vi "Example3.vi"() -> ()   [LabVIEW 2020]
doc: "Example of using propety node by direct and by reference."
panel:
  in  "stop":bool
  in  "Range":i32=2 format="%_1f"
  out "XY Graph":cluster{dbl[], dbl[]}[](graph)
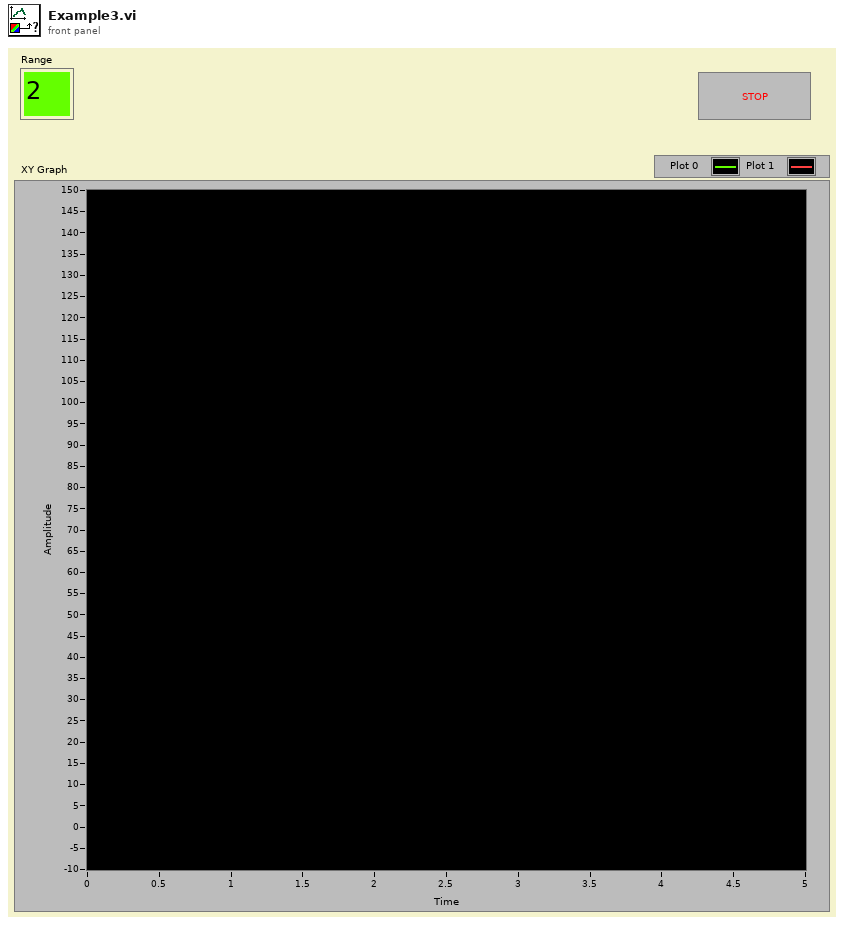
[diagram p1: front panel]
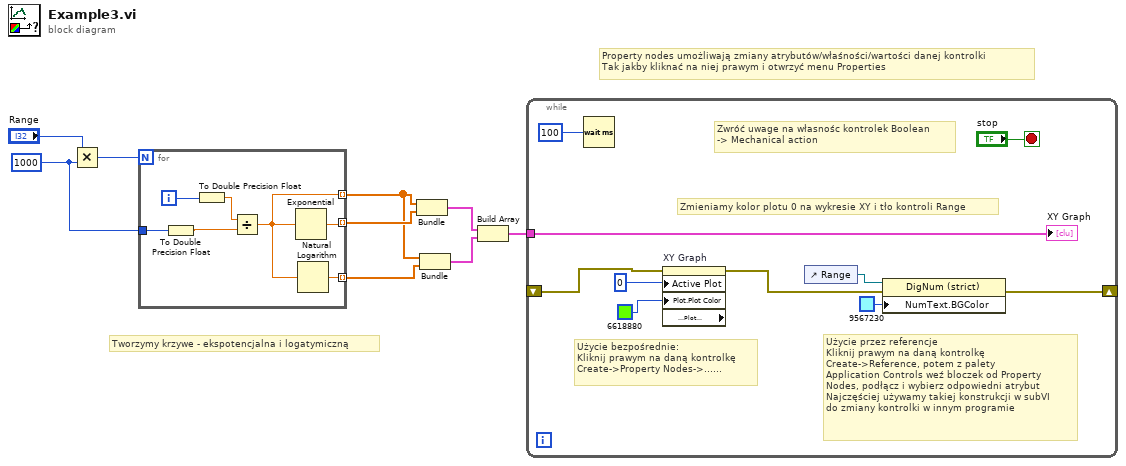
[diagram p0: block diagram]
diagram:
  w3 = 1000
  # "Tworzymy krzywe - ekspotencjalna i logatymiczną"
  # "Property nodes umożliwają zmiany atrybutów/właśności/wartości danej kontrolki \nTak jakby kliknać na niej prawym i otwrzyć menu Properties"
  n1 = Multiply(x="Range", y=w3) -> (x*y=w1:i32)
  n2 = for {
    N: w1 -> [_]
    tunnel: [w15] -> w9 mode=indexing
    tunnel: [w14] -> w8 mode=indexing
    tunnel: [w13] -> w7 mode=indexing
    tunnel: w3 -> [w11]
    i -> [w12]
    n3 = To Double Precision Float(number=w11) -> (double precision float=w10:dbl)
    n4 = To Double Precision Float(number=w12) -> (double precision float=w16:dbl)
    n5 = Divide(x=w16, y=w10) -> (x/y=w14:dbl)
    n6 = Exponential(1:w14) -> (0:w15:dbl)
    n7 = Natural Logarithm(1:w14) -> (0:w13:dbl)
  }
  n8 = Bundle(w8, w9) -> (w6:cluster{dbl[], dbl[]})  [unwired: 1 in]
  n9 = Bundle(w8, w7) -> (w5:cluster{dbl[], dbl[]})  [unwired: 1 in]
  n10 = Build Array(w6, w5) -> (w4:cluster{dbl[], dbl[]}[])
  n11 = while {
    tunnel: w4 -> [w26]
    shift-right: [w18] -> _
    shift-left: _ -> [w17]
    stop <- "stop" stop-if-true
    # "Zmieniamy kolor plotu 0 na wykresie XY i tło kontroli Range"
    # "Zwróć uwage na własnośc kontrolek Boolean\n-> Mechanical action"
    # "Użycie przez referencje\nKliknij prawym na daną kontrolkę \nCreate->Reference, potem z palety \nApplication Controls weź bloczek od Property\nNodes, podłącz i wybierz odpowiedni atrybut\nNajczęściej używamy takiej konstrukcji w subVI \ndo zmiany kontrolki w innym programie"
    # "Użycie bezpośrednie:\nKliknij prawym na daną kontrolkę \nCreate->Property Nodes->......"
    n12 = Wait (ms)(milliseconds to wait=u32 100) -> ()  [unwired: 1 out]
    n13 = property on="XY Graph" class="XYGraph (strict)" props=["Active Plot", "Plot", "Plot Color", "Plot", "Plot Interpolation"](error in=w17, "Active Plot"=u32 0, "Plot.Plot Color"=u32 6618880) -> (error out=w19:errorcluster)  [unwired: 1 in, 2 out]
    n14 = control-ref of="Range"() -> (w22:refnum<vi>)
    n15 = property class="DigNum (strict)"(reference=w22, error in=w19, "NumText.BGColor"=u32 9567230 ("Numeric Text.Text Colors:BG Color")) -> (error out=w18:errorcluster)  [unwired: 1 out]
    "XY Graph" <- w26
  }
